vi "Read_Write_Calibrations_Files.vi"   [LabVIEW 2018]
uses:
  <vilib>/Rock Robotics/Network Tables/NT Read String.vi
  <vilib>/Rock Robotics/Network Tables/NT Write String.vi
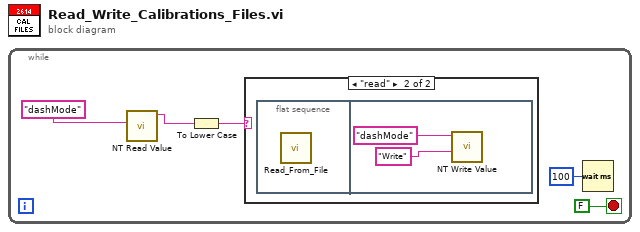
[diagram p0: block diagram]
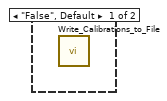
[diagram p2: hidden frame]
diagram:
  n1 = while {
    stop <- FALSE stop-if-true
    n2 = call-poly <vilib>:"NT Read Value.vi"("Name"="dashMode") -> ("String"=w1:string)  [unwired: 9 in, 1 out]
    n3 = To Lower Case(string=w1) -> (all lower case string=w2:string)
    n4 = case shown="\"read\"" w2 {
      frame "False", Default {
        n5 = call "Write_Calibrations_to_File.vi"() -> ()  [unwired: 12 in]
      }
      frame "read" {
        n6 = flat-sequence {
          frame #0 {
            n7 = call "Read_From_File.vi"() -> ()  [unwired: 12 in]
          }
          frame #1 {
            n8 = call-poly <vilib>:"NT Write Value.vi"("String"="Write", "Name"="dashMode") -> ()  [unwired: 9 in, 1 out]
          }
        }
      }
    }
    n9 = Wait (ms)(milliseconds to wait=u32 100) -> ()  [unwired: 1 out]
  }
